vi "Write Connected_.vi"(8 "error in (no error)":errorcluster, 10 "Connected?":bool, 11 "Realsense Cam in":refnum<class "Realsense Cam.lvclass">) -> (0 "error out":errorcluster, 3 "Realsense Cam out":refnum<class "Realsense Cam.lvclass">)   [LabVIEW 2018, in "Realsense Cam.lvclass"]
uses:
  Realsense Cam.lvclass
  Realsense Cam.lvclass/Realsense Cam.ctl
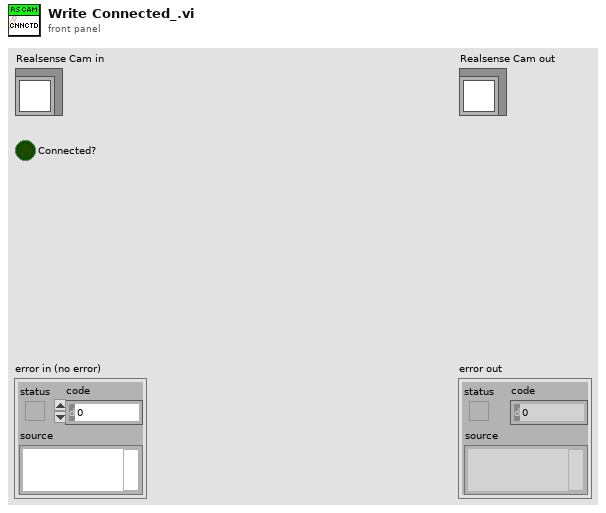
[diagram p1: front panel]
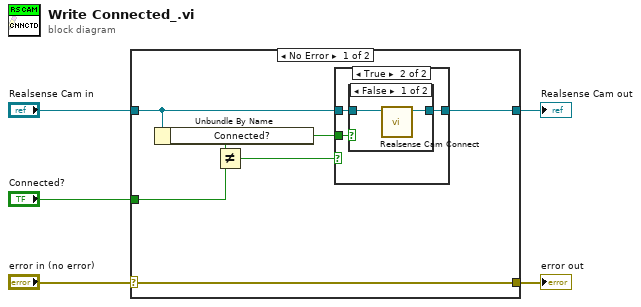
[diagram p0: block diagram]
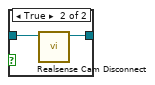
[diagram p3: hidden frame]
diagram:
  n1 = case shown="No Error" "error in (no error)" {
    selector: "error in (no error)" -> [w11 w20]
    tunnel: [w11 w20] -> w4
    tunnel: [w6 w21] -> w2
    tunnel: "Realsense Cam in" -> [w7 w21]
    tunnel: "Connected?" -> [w10 _]
    frame No Error {
      n2 = Unbundle By Name(w7) -> ("Connected?"=w8:bool)
      n3 = Not Equal?(x=w8, y=w10) -> (x != y?=w9:bool)
      n4 = case shown="True" w9 {
        tunnel: w8 -> [_ w15]
        tunnel: w7 -> [w12 w14]
        tunnel: [w12 w13] -> w6
        frame False {
        }
        frame True {
          n5 = case shown="False" w15 {
            tunnel: w14 -> [w17 w19]
            tunnel: [w16 w18] -> w13
            frame False {
              n6 = call-dynamic "Realsense Cam Connect.vi"("Realsense Cam In"=w17) -> ("Realsense Cam Out"=w16:refnum<class "Realsense Cam.lvclass">)  [unwired: 7 in, 3 out]
            }
            frame True {
              n7 = call-dynamic "Realsense Cam Disconnect.vi"("Realsense Cam in"=w19) -> ("Realsense Cam out"=w18:refnum<class "Realsense Cam.lvclass">)  [unwired: 8 in, 2 out]
            }
          }
        }
      }
    }
    frame Error {
    }
  }
  "error out" <- w4
  "Realsense Cam out" <- w2
